vi "zi-read.vi"(8 "error in (no error)":errorcluster, 11 "ZI Lockin in":refnum<class "ZI Lockin.lvclass">) -> (0 "error out":errorcluster, 2 "Result":dbl[](array[numeric]), 3 "ZI Lockin out":refnum<class "ZI Lockin.lvclass">)   [LabVIEW 2018, in "ZI Lockin.lvclass"]
uses:
  ZI Lockin.lvclass
  Users/Shared/github/NHMFL_Core/Libraries/Instruments/Instrument Driver/Instrument Driver.lvclass
  resonant_ultrasound_arxiv/maglab ultrasound -- arkady --arxiv/publisher action.ctl
  NHMFL_Core/Libraries/Instruments/Instrument Driver/Instrument Driver.lvclass/Instrument Driver.ctl
  Read ZI Handle.vi
  Write ZI Handle.vi
  NHMFL_Core/Libraries/Instruments/Instrument Driver/Write Channel names.vi
  NHMFL_Core/Libraries/Instruments/Instrument Driver/Write Channel units.vi
  <instrlib>/Zurich Instruments LabOne/Zurich Instruments LabOne.lvlib
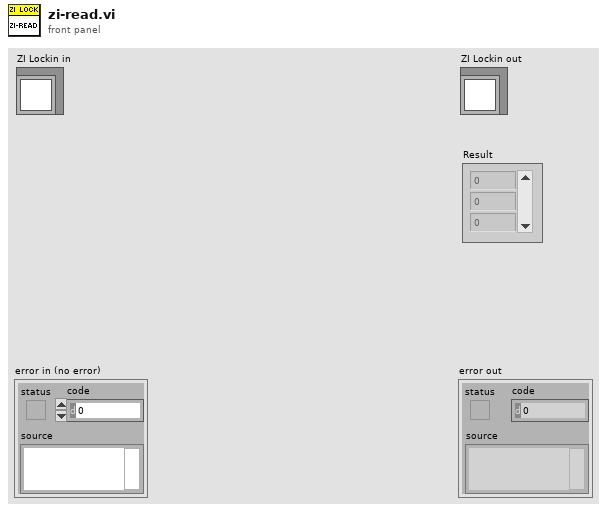
[diagram p1: front panel]
types:
  T1 = typedef "publisher action.ctl" = enum16{"set", "get"}
  T2 = typedef "Zurich Instruments LabOne.lvlib/ziTypeHandle.ctl" = cluster{"handleValid":bool, "Conn":u64, "Path Prefix":string, "Handle":u64, "Connected":bool, "Clockbase(s)":dbl}
  T3 = typedef "Zurich Instruments LabOne.lvlib/ziTypeDemodSampleSingle.ctl" = cluster{"Timestamps (ticks)":u64, "X (Vrms)":dbl, "Y (Vrms)":dbl, "Osc Phase (deg)":dbl, "Freq (Hz)":dbl, "DIO":u32, "AuxIn0 (V)":dbl, "AuxIn1 (V)":dbl, "Trigger":u32}
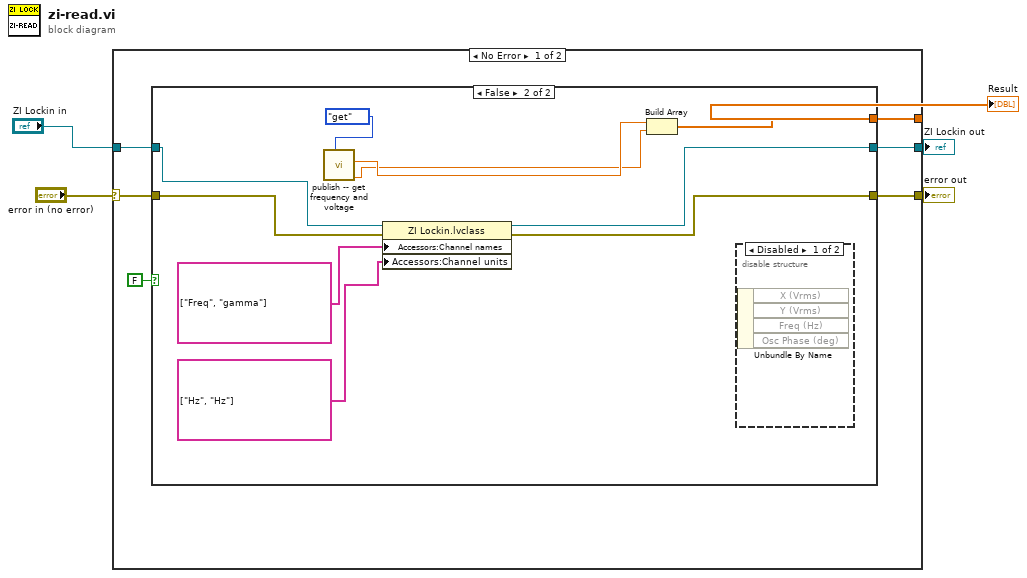
[diagram p0: block diagram]
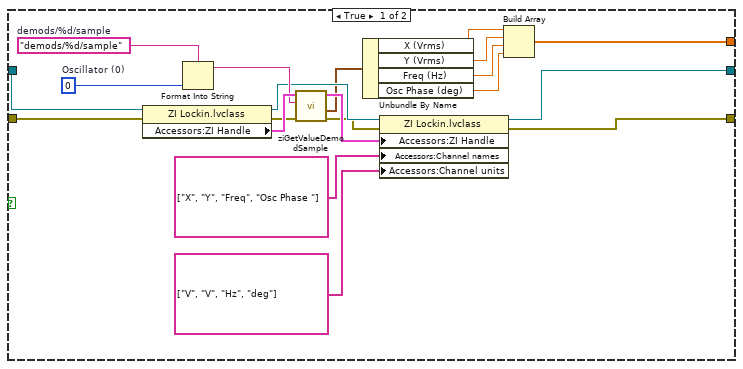
[diagram p2: hidden frame]
diagram:
  n1 = case shown="No Error" "error in (no error)" {
    selector: "error in (no error)" -> [w8 w43]
    tunnel: [w7 w43] -> w4
    tunnel: [w9 w42] -> w2
    tunnel: "ZI Lockin in" -> [w10 w42]
    tunnel: [w11 _] -> w1
    frame No Error {
      n2 = case shown="False" FALSE {
        tunnel: [w18 w41] -> w11
        tunnel: w10 -> [w17 w39]
        tunnel: [w16 w37] -> w9
        tunnel: w8 -> [w15 w36]
        tunnel: [w14 w35] -> w7
        frame True {
          w29 = u16 0  # Oscillator (0)
          w30 = "demods/%d/sample"  # demods/%d/sample
          n3 = property class="ZI Lockin.lvclass"(reference=w17, error in=w15) -> (reference out=w26:refnum<class "ZI Lockin.lvclass">, error out=w27:errorcluster, "Accessors:ZI Handle"=w31:T2)
          n4 = Format Into String(format string=w30, w29) -> (resulting string=w28:string)  [unwired: 2 in, 1 out]
          n5 = call <instrlib>:"ziGetValueDemodSample.vi"("error in"=w27, "Path"=w28, "Handle In"=w31) -> ("error out"=w24:errorcluster, "Demod Sample Out"=w23:T3, "Handle Out"=w25:T2)  [unwired: 2 in]
          n6 = Unbundle By Name(w23) -> ("X (Vrms)"=w22:dbl, "Y (Vrms)"=w21:dbl, "Freq (Hz)"=w20:dbl, "Osc Phase (deg)"=w19:dbl)
          n7 = property class="ZI Lockin.lvclass"(reference=w26, error in=w24, "Accessors:ZI Handle"=w25, "Accessors:Channel names"=string[] ["X", "Y", "Freq", "Osc Phase "] ("Channel names"), "Accessors:Channel units"=string[] ["V", "V", "Hz", "deg"] ("Channel names")) -> (reference out=w16:refnum<class "ZI Lockin.lvclass">, error out=w14:errorcluster)
          n8 = Build Array(w22, w21, w20, w19) -> (w18:dbl[])
        }
        frame False {
          n9 = call "publish -- get frequency and voltage.vi"("publisher action"=publisher_action."get") -> ("gamma OUT (Hz)"=w32:dbl, "freq out (Hz)"=w33:dbl)  [unwired: 8 in, 1 out]
          n10 = property class="ZI Lockin.lvclass"(reference=w39, error in=w36, "Accessors:Channel names"=string[] ["Freq", "gamma"] ("Channel names"), "Accessors:Channel units"=string[] ["Hz", "Hz"] ("Channel names")) -> (reference out=w37:refnum<class "ZI Lockin.lvclass">, error out=w35:errorcluster)
          n11 = Build Array(w33, w32) -> (w41:dbl[])
          n12 = disable-structure shown="Disabled" {
            frame Disabled {
              n13 = Unbundle By Name() -> ()  [unwired: 1 in, 4 out]
            }
            frame Enabled {
            }
          }
        }
      }
    }
    frame Error {
    }
  }
  "error out" <- w4
  "ZI Lockin out" <- w2
  "Result" <- w1
